vi "Get Parent.vi"(0 "Tree Reference In":refnum<vi>, 2 "Child Tag (Current)":string, 5 "error in (no error)":errorcluster) -> (14 "Tree Reference Out":refnum<vi>, 16 "Parent Tag":string, 17 "Parents Tags":string[](array[string]), 19 "error out":errorcluster)   [LabVIEW 2010]
doc: "Retrieves the parent of the child. Uses the currently selected item if input is left unwired or empty string. Also returns a 1-D array of all members in its family starting at its parent and leading back to its most mature member."
panel:
  # "VI INPUTS"
  # "VI OUTPUTS"
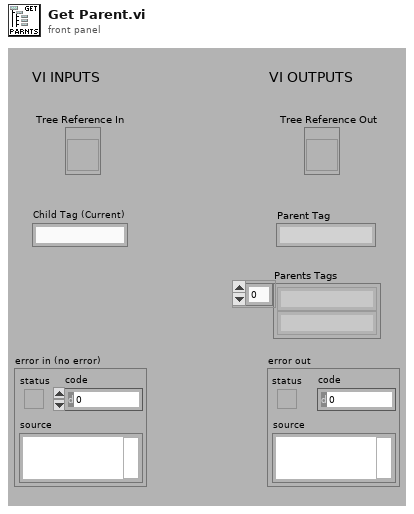
[diagram p1: front panel]
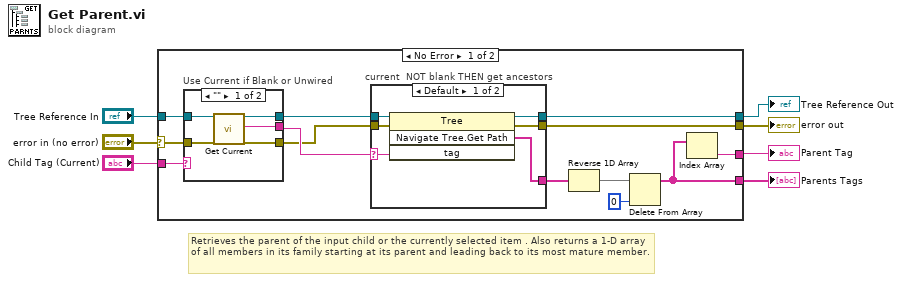
[diagram p0: block diagram]
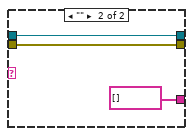
[diagram p3: hidden frame]
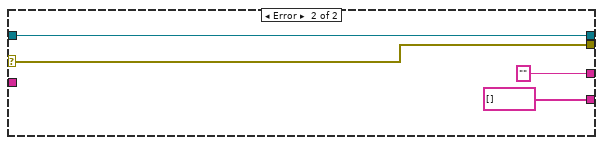
[diagram p4: hidden frame]
diagram:
  # "Retrieves the parent of the input child or the currently selected item . Also returns a 1-D array of all members in its family starting at its parent and leading back to its most mature member."
  n1 = case shown="No Error" "error in (no error)" {
    selector: "error in (no error)" -> [w17 w40]
    tunnel: "Tree Reference In" -> [w18 w41]
    tunnel: "Child Tag (Current)" -> [w16 _]
    tunnel: [w20 w41] -> w5
    tunnel: [w8 string[] []] -> w4
    tunnel: [w19 w40] -> w3
    tunnel: [w12 ""] -> w1
    frame No Error {
      n2 = case "Use Current if Blank or Unwired" shown="\"\"" w16 {
        selector: w16 -> [_ w26]
        tunnel: [w24 w28] -> w13
        tunnel: w18 -> [w25 w28]
        tunnel: [w23 w27] -> w14
        tunnel: w17 -> [w22 w27]
        tunnel: [w21 w26] -> w15
        frame "" {
          n3 = call <userlib>:"Get Current.vi"("Tree Reference In"=w25, "error in (no error)"=w22) -> ("Tree Reference Out"=w24:refnum<vi>, "Current Tag"=w21:string, "error out"=w23:errorcluster)  [unwired: 14 in, 1 out]
        }
        frame Default {
        }
      }
      n4 = case "current  NOT blank THEN get ancestors" shown="Default" w15 {
        selector: w15 -> [w29 _]
        tunnel: w13 -> [w34 w37]
        tunnel: [w33 w36] -> w19
        tunnel: [w30 string[] [] ("Navigate Tree:Get Path")] -> w10
        tunnel: [w32 w37] -> w20
        tunnel: w14 -> [w31 w36]
        frame Default {
          n5 = invoke class="Tree" method="Navigate Tree.Get Path"(reference=w34, error in=w31, "tag"=w29) -> (reference out=w32:refnum<vi>, error out=w33:errorcluster, "Navigate Tree:Get Path"=w30:string[])  [unwired: 1 in, 1 out]
        }
        frame "" {
        }
      }
      n6 = Reverse 1D Array(array=w10) -> (reversed array=w9:string[])
      n7 = Delete From Array(array=w9, index=0) -> (array with subset deleted=w8:string[])  [unwired: 1 in, 1 out]
      n8 = Index Array(array=w8) -> (element=w12:string)  [unwired: 1 in]
    }
    frame Error {
    }
  }
  "Parents Tags" <- w4
  "Tree Reference Out" <- w5
  "error out" <- w3
  "Parent Tag" <- w1
